vi "___set_field_current.vi"(2 "Yokogawa Address":refnum<visa-resource-name>="GPIB0::25::INSTR", 3 "error in":errorcluster, 5 "I mA":dbl=0.2362 step=2e-05) -> (0 "error out":errorcluster)   [LabVIEW 2013]
uses:
  present_current.vi
panel:
  out "resulting string":string
  out "Out of range":bool
  out "Present I (mA)":dbl=0.2362
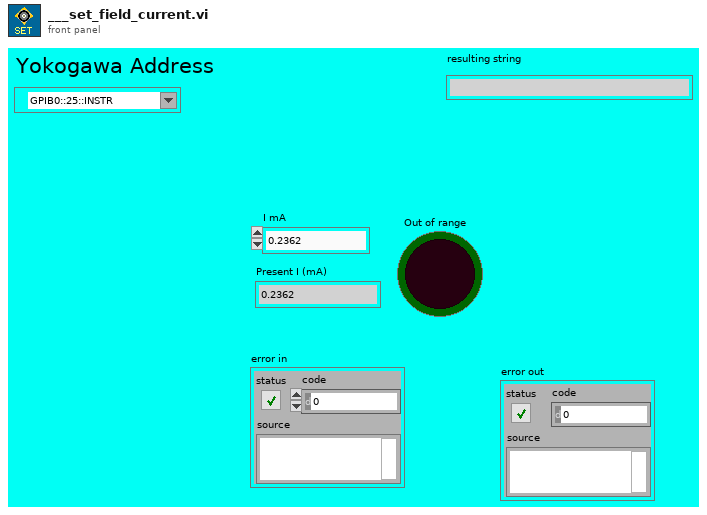
[diagram p1: front panel]
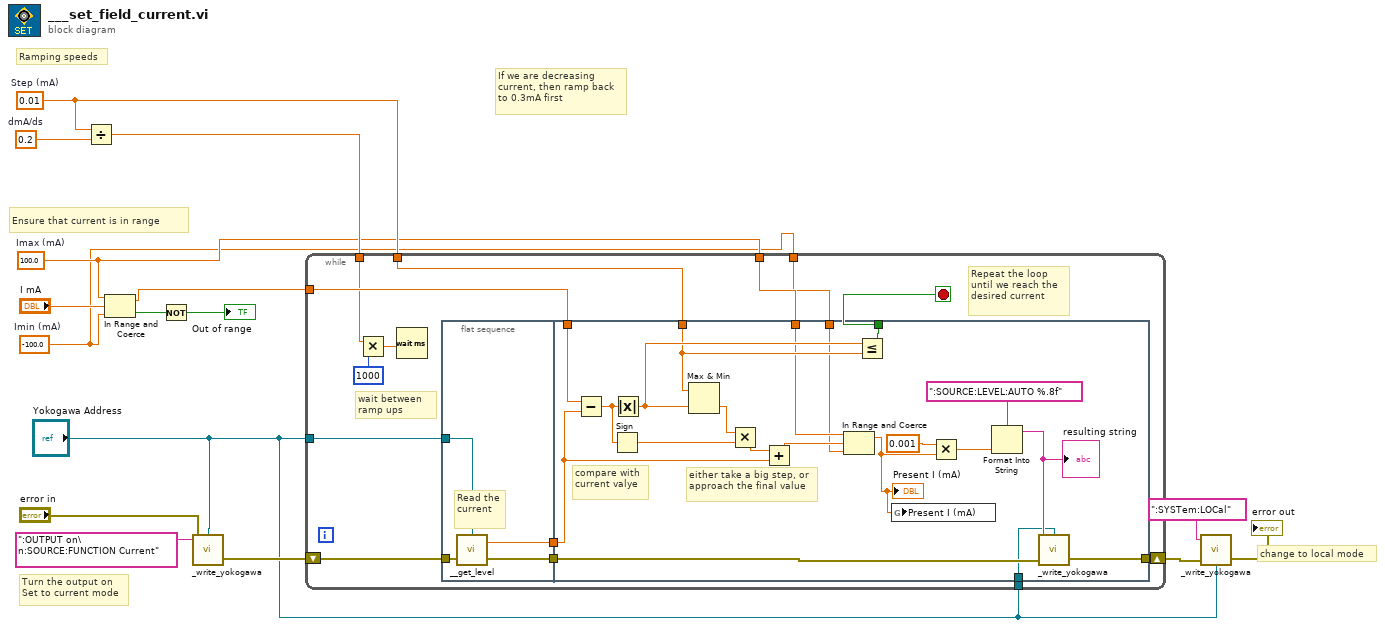
[diagram p0: block diagram]
diagram:
  w15 = 0.2  # dmA/ds
  w12 = 0.01  # Step (mA)
  w7 = 100.0  # Imax (mA)
  w6 = -100.0  # Imin (mA)
  # "Ramping speeds"
  # "If we are decreasing\ncurrent, then ramp back\nto 0.3mA first"
  # "change to local mode"
  # "Ensure that current is in range"
  # "Turn the output on\nSet to current mode"
  n1 = Divide(x=w12, y=w15) -> (x/y=w14:dbl)
  n2 = In Range and Coerce(upper limit=w7, x="I mA", lower limit=w6) -> (coerced(x)=w5:dbl, In Range?=w9:bool)
  n3 = Not(x=w9) -> (.not. x?=→"Out of range":bool)
  n4 = call "_write_yokogawa.vi"("Yokogawa Address"="Yokogawa Address", "error in"="error in", "write buffer"=":OUTPUT on\n:SOURCE:FUNCTION Current") -> ("error out"=w4:errorcluster)  [unwired: 2 in]
  n5 = while {
    tunnel: w14 -> [w23]
    tunnel: w12 -> [w26]
    tunnel: w5 -> [w27]
    shift-right: [w21] -> w11
    shift-left: w4 -> [w28]
    tunnel: w7 -> [w20]
    tunnel: w6 -> [w19]
    tunnel: "Yokogawa Address" -> [w18]
    tunnel: "Yokogawa Address" -> [w17]
    stop <- w30 stop-if-true
    # "wait between ramp ups"
    # "Repeat the loop until we reach the desired current"
    n6 = Multiply(x=w23, y=1000) -> (x*y=w24:dbl)
    n7 = Wait (ms)(milliseconds to wait=w24) -> ()  [unwired: 1 out]
    n8 = flat-sequence {
      tunnel: [w33] -> w29
      tunnel: w28 -> [w34]
      tunnel: [w32] -> w22
      tunnel: w18 -> [w31]
      tunnel: [w46] -> w30
      tunnel: w29 -> [w48]
      tunnel: w27 -> [w42]
      tunnel: w26 -> [w41]
      tunnel: w22 -> [w40]
      tunnel: [w39] -> w21
      tunnel: w20 -> [w38]
      tunnel: w19 -> [w37]
      tunnel: w17 -> [w35]
      frame #0 {
        # "Read the \ncurrent"
        n9 = call "__get_level.vi"("Yokogawa Address"=w31, "error in"=w34) -> ("error out"=w32:errorcluster, "Current (mA)"=w33:dbl)  [unwired: 2 in]
      }
      frame #1 {
        # "either take a big step, or approach the final value"
        # "compare with current valye"
        n10 = Subtract(x=w42, y=w48) -> (x-y=w49:dbl)
        n11 = Sign(1:w49) -> (0:w51:dbl)
        n12 = Absolute Value(x=w49) -> (abs(x)=w47:dbl)
        n13 = Max & Min(x=w41, y=w47) -> (min(x,y)=w52:dbl)  [unwired: 1 out]
        n14 = Multiply(x=w52, y=w51) -> (x*y=w50:dbl)
        n15 = Add(x=w50, y=w48) -> (x+y=w53:dbl)
        n16 = In Range and Coerce(upper limit=w38, x=w53, lower limit=w37) -> (coerced(x)=w36:dbl)  [unwired: 1 out]
        "Present I (mA)" <- w36
        n17 = Less Or Equal?(x=w47, y=w41) -> (x <= y?=w46:bool)
        n18 = global write "present_current.vi" "Present I (mA)"(w36) -> ()
        n19 = Multiply(x=0.001, y=w36) -> (x*y=w44:dbl)
        n20 = Format Into String(format string=":SOURCE:LEVEL:AUTO %.8f", w44) -> (resulting string=w43:string)  [unwired: 2 in, 1 out]
        "resulting string" <- w43
        n21 = call "_write_yokogawa.vi"("Yokogawa Address"=w35, "error in"=w40, "write buffer"=w43) -> ("error out"=w39:errorcluster)  [unwired: 2 in]
      }
    }
  }
  n22 = call "_write_yokogawa.vi"("Yokogawa Address"="Yokogawa Address", "error in"=w11, "write buffer"=":SYSTem:LOCal") -> ("error out"=→"error out":errorcluster)  [unwired: 2 in]
